vi "raster-scanning_simplify.vi"() -> ()   [LabVIEW 2017]
uses:
  raster-scan-params.ctl
  controls/PI-params.ctl
  controls/boolean_info.ctl
  <vilib>/rvi/Emulation/niFpgaGetClockAttributes.vi
  <vilib>/rvi/Emulation/niFpgaSctlEmulationGetInTimedLoop.vi
  <vilib>/rvi/Emulation/niFpgaEmulationReportErrorSimple.vi
  <vilib>/rvi/eio/common/nirviEmuTemplateMethod_errors.vi
  <vilib>/rvi/Emulation/niFpgaEmulationIsFPGAContextNoSignature.vi
  <vilib>/rvi/DataTransferAndStorage/Container/Common/niFpgaContainerGetUniqueNameForEmu.vi
  <vilib>/rvi/Memory/Memory_Emulation/niFpgaMemoryEmulationCacheClearOnFirstRun.vi
  <vilib>/rvi/Memory/Memory_Emulation/nirvimemoryEmulationManagerCache_MakeExclusive.vi
  <vilib>/rvi/Memory/Memory_Emulation/niFpgaMemoryEmulationValidateCache.vi
  <vilib>/rvi/Memory/Memory_Emulation/nirvimemoryEmulationManagerCache_InsertValue.vi
  <vilib>/Utility/error.llb/Clear Errors.vi
  <vilib>/rvi/Memory/Memory_Emulation/nirvimemoryEmulationManagerCache_ReleaseExclusive.vi
  <vilib>/rvi/Memory/Memory_Emulation/nirvimemoryEmulationManagerCache_GetValue.vi
  <vilib>/rvi/Memory/Memory_Emulation/nirvimemoryEmulationManagerCache_SetValue.vi
  <vilib>/rvi/Emulation/niFpgaProcessEmulError.vi
  <vilib>/rvi/DataTransferAndStorage/Container/Common/niFpgaContainerExecOnDevCompGetState.vi
  <vilib>/rvi/Emulation/niFpgaCriticalErrorInLSC.vi
  <vilib>/eio/EIONode/EIONode.xnode
  <vilib>/rvi/DataTransferAndStorage/Container/XNode/niFpgaContainer.xnode
  <vilib>/rvi/DataTransferAndStorage/Register/Emulation/niFpgaRegisterEmulation.vi
  <vilib>/rvi/DataTransferAndStorage/Register/Emulation/niFpgaRegisterEmulationRefIn.vi
  libimaging-cs.lvlib
  FPGA-data-logging.lvlib
panel:
  out "boolean errors":T1
  in  "xy-init":fxp<+/-,16,5>[](array[numeric])=[0.0, 0.0]
  in  "Ki-xy":sgl=0.001 format="%#_13g"
  in  "xy-bound":sgl
  in  "trigger-0":bool
  in  "u(0)":sgl format="%#_13g"
  out "e(0) (threshhold init)":fxp<+/-,16,5>
  out "current-case":i16
  out "DAC-zaxis":sgl
  out "ADC-zaxis":fxp<+/-,24,5>
  in  "raise-constant":sgl
  in  "raster-scan-params":T2={"TsTicks"=1600, "Stop"=TRUE, "TOL"=0.3, "ramp-rate"=0.0, "z-u-max"=5.0, "PI-params"={"Ki"=0.001, "setpoint"=0.0}, "Num"=[-0.00254, 0.000408, 0.00295, 0.0, 0.0, 0.0, 0.0, 0.0, 0.0], "TF Order"=2, "Den"=[0.982758, -1.98194, 1.0, 0.0, 0.0, 0.0, 0.0, 0.0, 0.0]} {"z-u-max" format="%#_13g"; "TOL" format="%#_13g"}
  # "DIAGNOSTICS"
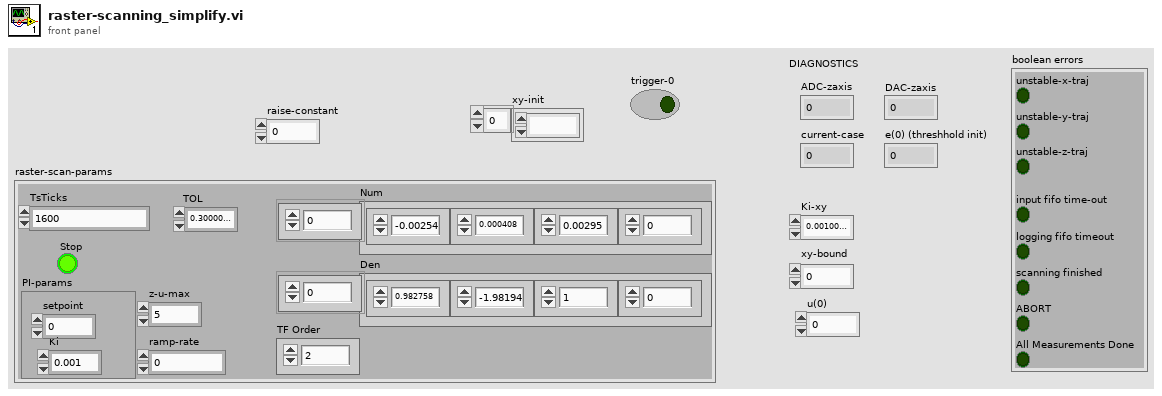
[diagram p1: front panel]
types:
  T1 = typedef "boolean_info.ctl" = cluster{"unstable-z-traj":bool, "input fifo time-out":bool, "logging fifo timeout":bool, "scanning finished":bool, "unstable-x-traj":bool, "unstable-y-traj":bool, "ABORT":bool, "All Measurements Done":bool}
  T2 = typedef "raster-scan-params.ctl" = cluster{"TsTicks":u32, "Stop":bool, "TOL":sgl, "ramp-rate":sgl, "z-u-max":sgl, "PI-params":T3, "Num":sgl[], "TF Order":i32, "Den":sgl[]}
  T3 = typedef "PI-params.ctl" = cluster{"Ki":sgl, "setpoint":sgl}
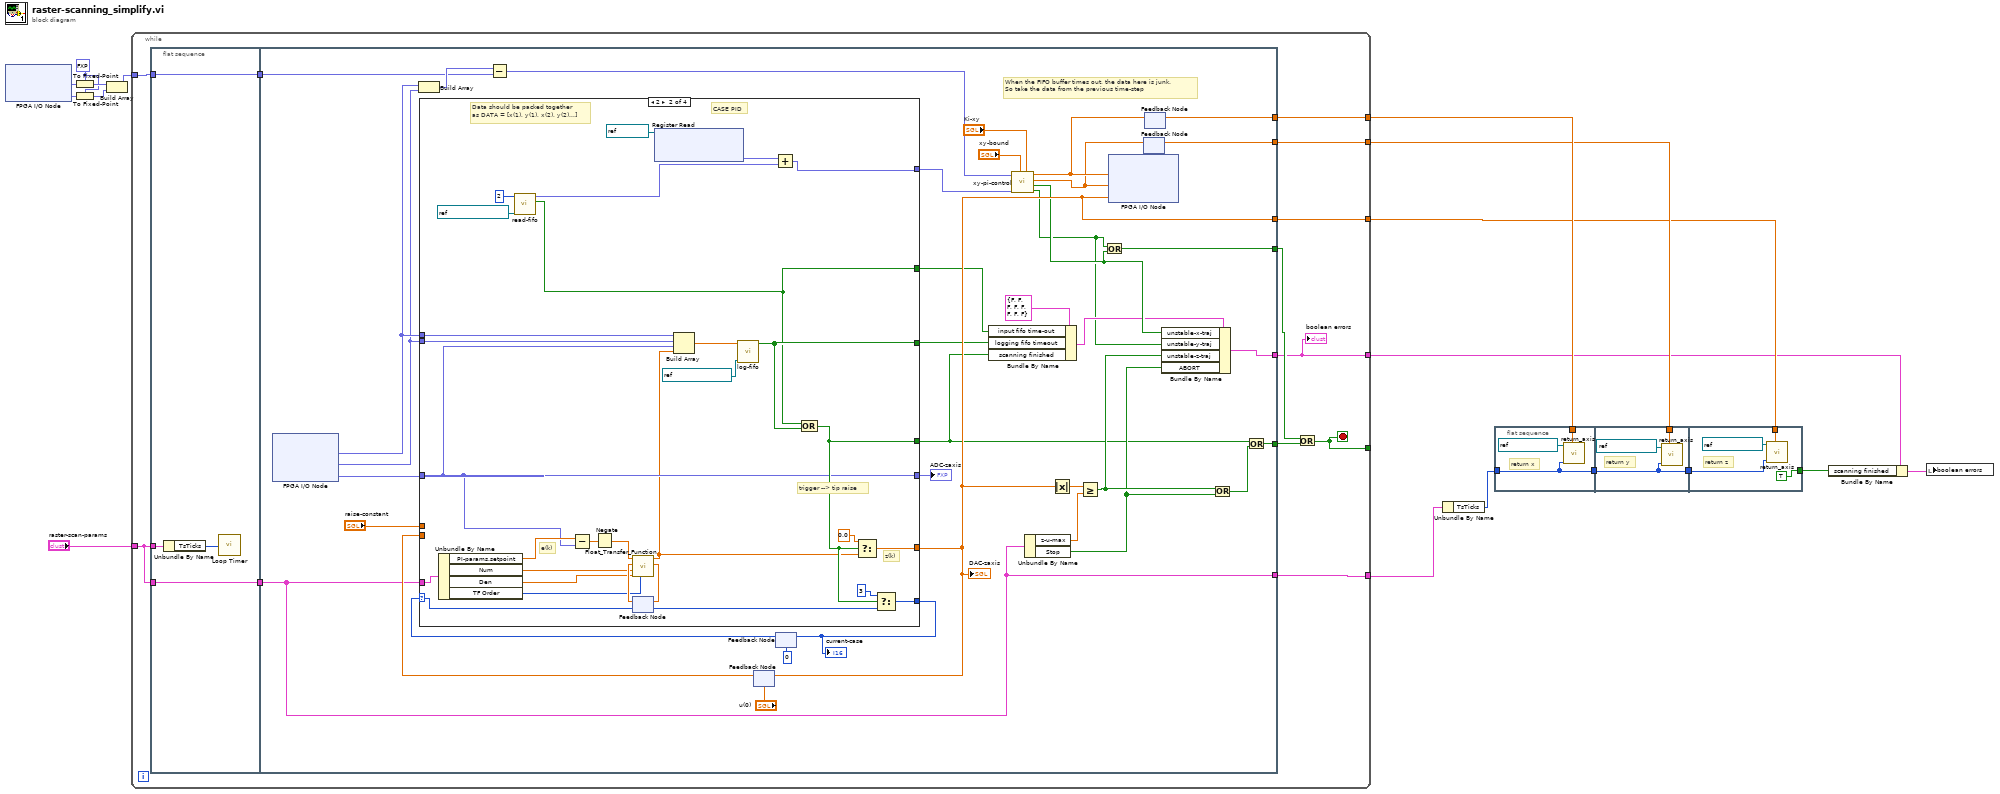
[diagram p0: block diagram]
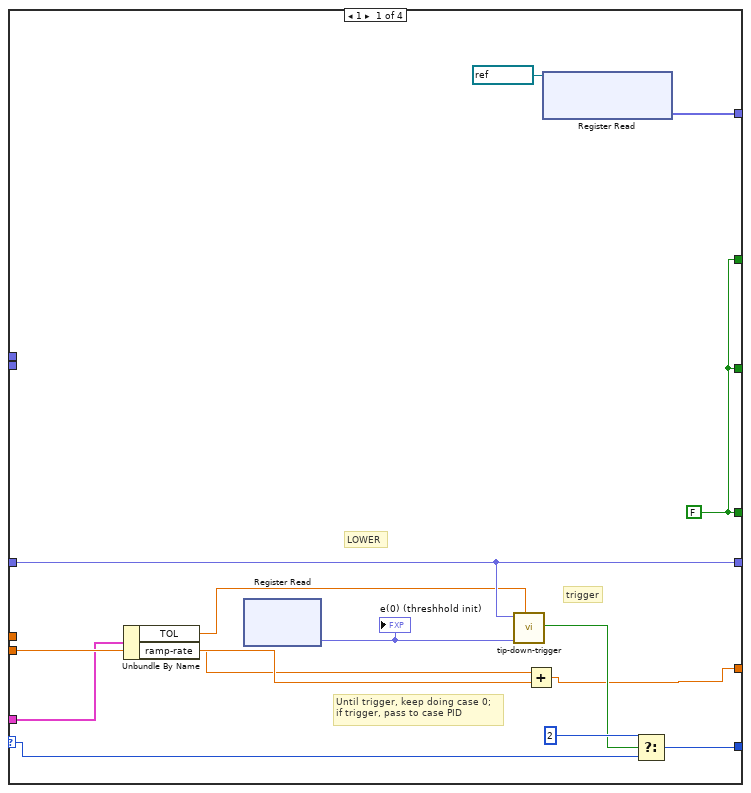
[diagram p2: hidden frame]
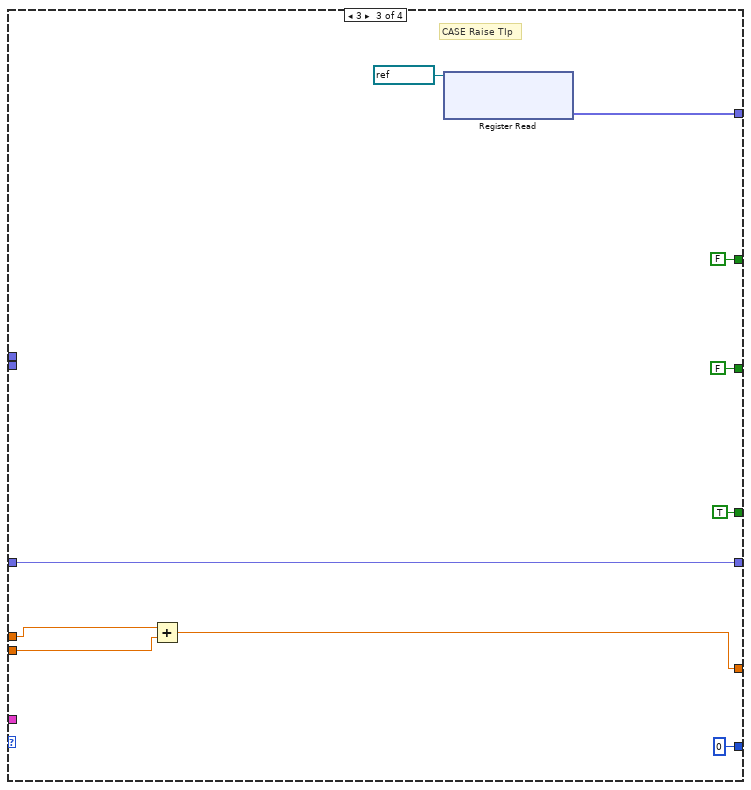
[diagram p3: hidden frame]
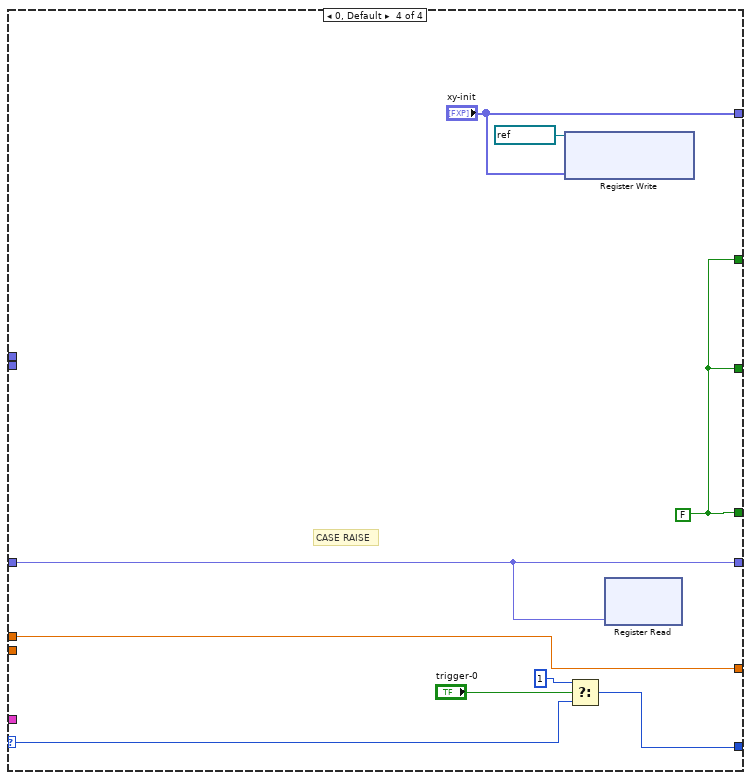
[diagram p4: hidden frame]
diagram:
  w2 = fxp<+/-,16,5> 0.0 ("fixed-point type")
  n1 = xnode "FPGA I/O Node"() -> ("Mod2/AI0"=w5:fxp<+/-,24,5>, "Mod2/AI1"=w3:fxp<+/-,24,5>)  [unwired: 2 in, 2 out]
  n2 = To Fixed-Point(fixed-point type=w2, number=w5) -> (fixed-point=w6:fxp<+/-,16,5>)
  n3 = To Fixed-Point(fixed-point type=w2, number=w3) -> (fixed-point=w4:fxp<+/-,16,5>)
  n4 = Build Array(w6, w4) -> (w1:fxp<+/-,16,5>[])
  n5 = while {
    tunnel: [w22] -> _
    tunnel: "raster-scan-params" -> [w28]
    tunnel: [w27] -> w16
    tunnel: [w26] -> w14
    tunnel: [w20] -> w8
    tunnel: [w25] -> w12
    tunnel: [w24] -> w13
    tunnel: w1 -> [w18]
    stop <- w22 stop-if-true
    n6 = flat-sequence {
      tunnel: w28 -> [w32]
      tunnel: [w31] -> w29
      tunnel: w28 -> [w31]
      tunnel: w18 -> [w30]
      tunnel: [w30] -> w19
      tunnel: [w65] -> w23
      tunnel: w29 -> [w60]
      tunnel: [w59] -> w26
      tunnel: [w60] -> w27
      tunnel: [w56] -> w20
      tunnel: [w46] -> w25
      tunnel: [w49] -> w24
      tunnel: [w45] -> w21
      tunnel: w19 -> [w41]
      frame #0 {
        n7 = Unbundle By Name(w32) -> ("TsTicks"=w33:u32)
        n8 = call "Loop Timer"("Count(Ticks)"=w33) -> ()  [unwired: 1 out]
      }
      frame #1 {
        # "When the FIFO buffer times out, the data here is junk.\nSo take the data from the previous time-step"
        n9 = xnode "FPGA I/O Node"() -> ("Mod2/AI0"=w53:fxp<+/-,24,5>, "Mod2/AI1"=w52:fxp<+/-,24,5>, "Mod2/AI2"=w70:fxp<+/-,24,5>)  [unwired: 3 in, 3 out]
        n10 = Build Array(w53, w52) -> (w42:fxp<+/-,24,5>[])
        n11 = Subtract(x=w42, y=w41) -> (x-y=w40:fxp<+/-,25,6>[])
        n12 = feedback #1("u(0)") -> (w64:sgl)
        n13 = feedback #2(i16 0 ("f")) -> (w66:i16)
        n14 = case shown="2" w66 {
          selector: w66 -> [w73 w106 _ w127]
          tunnel: w64 -> [w84 _ w122 _]
          tunnel: w70 -> [w81 w86 w116 w132]
          tunnel: [w81 w86 w116 w132] -> w69
          tunnel: [w83 w112 i16 0 ("f") w130] -> w67
          tunnel: w52 -> [_ w110 _ _]
          tunnel: w53 -> [_ w109 _ _]
          tunnel: [w74 w107 TRUE ("Timed Out?") w129] -> w39
          tunnel: [w78 w108 w121 w126] -> w46
          tunnel: w60 -> [w77 w87 _ _]
          tunnel: [w74 w100 FALSE ("Timed Out?") w129] -> w37
          tunnel: [w74 w104 FALSE ("Timed Out?") w129] -> w38
          tunnel: [w71 w97 w114 "xy-init"] -> w48
          tunnel: "raise-constant" -> [_ _ w123 w126]
          frame 1 {
            w74 = FALSE ("Timed Out?")
            # "Until trigger, keep doing case 0;\nif trigger, pass to case PID"
            # "LOWER"
            # "trigger"
            n15 = Unbundle By Name(w77) -> ("TOL"=w76:sgl, "ramp-rate"=w75:sgl)
            n16 = xnode ("Register Read")() -> ("Data"=w79:fxp<+/-,16,5>)  [unwired: 1 in, 1 out]
            "e(0) (threshhold init)" <- w79
            n17 = call "tip-down-trigger.vi"("TOL"=w76, "Vo"=w79, "e(k)"=w81) -> ("trigger"=w80:bool)  [unwired: 8 in]
            n18 = Add(x=w75, y=w84) -> (x+y=w78:sgl)
            n19 = xnode ("Register Read")("Register In"=refnum<k21> "xy_init") -> ("Data"=w71:fxp<+/-,17,6>[])  [unwired: 1 out]
            n20 = Select(t=i16 2, s=w80, f=w73) -> (s? t:f=w83:i16)
          }
          frame 2 {
            # "e(k)"
            # "Data should be packed together\nas DATA = [x(1), y(1), x(2), y(2)...]"
            # "trigger --> tip raise"
            # "z(k)"
            # "CASE PID"
            n21 = Unbundle By Name(w87) -> ("PI-params.setpoint"=w94:sgl, "Num"=w91:sgl[], "Den"=w90:sgl[], "TF Order"=w89:i32)
            n22 = call "read-fifo.vi"("FIFO In"=refnum<k21> "Host_to_FPGA", "numChan"=2) -> ("timout?"=w100:bool, "unpacked-data"=w96:fxp<+/-,16,5>[])  [unwired: 8 in]
            n23 = Subtract(x=w94, y=w86) -> (x-y=w95:sgl)
            n24 = Negate(x=w95) -> (-x=w88:sgl)
            n25 = feedback #3() -> (w92:sgl[])  [unwired: 1 in]
            n26 = call "Float_Transfer_Function.vi"("TF Order"=w89, "Den"=w90, "Num"=w91, "State In"=w92, "Input"=w88) -> ("State Out"=w93:sgl[], "Output"=w85:sgl)  [unwired: 4 in]
            n27 = feedback-in #3(w93) -> ()
            n28 = xnode ("Register Read")("Register In"=refnum<k21> "xy_init") -> ("Data"=w98:fxp<+/-,17,6>[])  [unwired: 1 out]
            n29 = Build Array(w109, w110, w86, w85) -> (w105:sgl[])
            n30 = call "log-fifo.vi"("FIFO In"=refnum<k21> "fpga-to-host2", "input-data"=w105) -> ("logging-timeout?"=w104:bool)  [unwired: 9 in]
            n31 = Add(x=w98, y=w96) -> (x+y=w97:fxp<+/-,18,7>[])
            n32 = Compound Arithmetic op=OR(w100, w104) -> (w107:bool)
            n33 = Select(t=sgl 0.0 ("f"), s=w107, f=w85) -> (s? t:f=w108:sgl)
            n34 = Select(t=i16 3, s=w107, f=w106) -> (s? t:f=w112:i16)
          }
          frame 3 {
            # "CASE Raise TIp"
            n35 = Add(x=w123, y=w122) -> (x+y=w121:sgl)
            n36 = xnode ("Register Read")("Register In"=refnum<k21> "xy_init") -> ("Data"=w114:fxp<+/-,17,6>[])  [unwired: 1 out]
          }
          frame 0, Default {
            w129 = FALSE ("Timed Out?")
            # "CASE RAISE"
            n37 = xnode ("Register Write")("Data"="xy-init", "Register In"=refnum<k21> "xy_init") -> ()  [unwired: 1 out]
            n38 = Select(t=i16 1 ("f"), s="trigger-0", f=w127) -> (s? t:f=w130:i16)
            n39 = xnode ("Register Read")("Data"=w132) -> ()  [unwired: 1 in, 1 out]
          }
        }
        "ADC-zaxis" <- w69
        "DAC-zaxis" <- w46
        "current-case" <- w67
        n40 = feedback-in #1(w46) -> ()
        n41 = feedback-in #2(w67) -> ()
        n42 = Bundle By Name(cluster=T1 {"unstable-z-traj"=FALSE, "input fifo time-out"=FALSE, "logging fifo timeout"=FALSE, "scanning finished"=FALSE, "unstable-x-traj"=FALSE, "unstable-y-traj"=FALSE, "ABORT"=FALSE, "All Measurements Done"=FALSE} ("boolean errors 2"), "input fifo time-out"=w37, "logging fifo timeout"=w38, "scanning finished"=w39) -> (w35:T1)
        n43 = call "xy-pi-control.vi"("Ki-xy"="Ki-xy", "xy-umax"="xy-bound", "xy-ref"=w48, "x_k-y_k"=w40) -> ("u_y saturated"=w34:bool, "u_x saturated"=w44:bool, "sat(u_y)"=w50:sgl, "sat(u_x)"=w51:sgl)  [unwired: 4 in]
        n44 = Unbundle By Name(w60) -> ("z-u-max"=w62:sgl, "Stop"=w57:bool)
        n45 = Absolute Value(x=w46) -> (abs(x)=w68:sgl)
        n46 = Greater Or Equal?(x=w68, y=w62) -> (x >= y?=w58:bool)
        n47 = Or(x=w34, y=w44) -> (x .or. y?=w45:bool)
        n48 = xnode "FPGA I/O Node"("Mod1/AO0"=w51, "Mod1/AO1"=w50, "Mod1/AO2"=w46) -> ()  [unwired: 3 in, 3 out]
        n49 = feedback #4() -> (w49:sgl)  [unwired: 1 in]
        n50 = feedback-in #4(w50) -> ()
        n51 = feedback-in #5(w51) -> ()
        n52 = feedback #5() -> (w59:sgl)  [unwired: 1 in]
        n53 = Bundle By Name(cluster=w35, "unstable-x-traj"=w44, "unstable-y-traj"=w34, "unstable-z-traj"=w58, "ABORT"=w57) -> (w56:T1)
        n54 = Or(x=w58, y=w57) -> (x .or. y?=w61:bool)
        n55 = Or(x=w39, y=w61) -> (x .or. y?=w65:bool)
      }
    }
    n56 = Or(x=w21, y=w23) -> (x .or. y?=w22:bool)
    "boolean errors" <- w20
  }
  n57 = Unbundle By Name(w16) -> ("TsTicks"=w15:u32)
  n58 = flat-sequence {
    tunnel: w15 -> [w134]
    tunnel: w14 -> [w135]
    tunnel: [w134] -> w11
    tunnel: w13 -> [w138]
    tunnel: w11 -> [w136]
    tunnel: [w136] -> w10
    tunnel: w12 -> [w142]
    tunnel: w10 -> [w140]
    tunnel: [TRUE] -> w9
    frame #0 {
      # "return x"
      n59 = call "return_axis.vi"("u(0)"=w135, "TsTicks"=w134, "FPGA I/O In"=refnum<k21> "Mod1/AO0") -> ()  [unwired: 9 in]
    }
    frame #1 {
      # "return y"
      n60 = call "return_axis.vi"("u(0)"=w138, "TsTicks"=w136, "FPGA I/O In"=refnum<k21> "Mod1/AO1") -> ()  [unwired: 9 in]
    }
    frame #2 {
      # "return z"
      n61 = call "return_axis.vi"("u(0)"=w142, "TsTicks"=w140, "FPGA I/O In"=refnum<k21> "Mod1/AO2") -> ()  [unwired: 9 in]
    }
  }
  n62 = Bundle By Name(cluster=w8, "scanning finished"=w9) -> (w7:T1)
  n63 = local write "boolean errors"(w7) -> ()
